vi "Set Node IDs.vi"(8 "error in (no error)":errorcluster, 10 "FolderIDs":T2, 11 "Station in":refnum<class "Station.lvclass">) -> (0 "error out":errorcluster, 3 "Station out":refnum<class "Station.lvclass">)   [LabVIEW 2021, in "Station.lvlib" / "Station.lvclass"]
uses:
  Station.lvclass
  <vilib>/OPCUA/controls/OPC UA Server Refnum.ctl
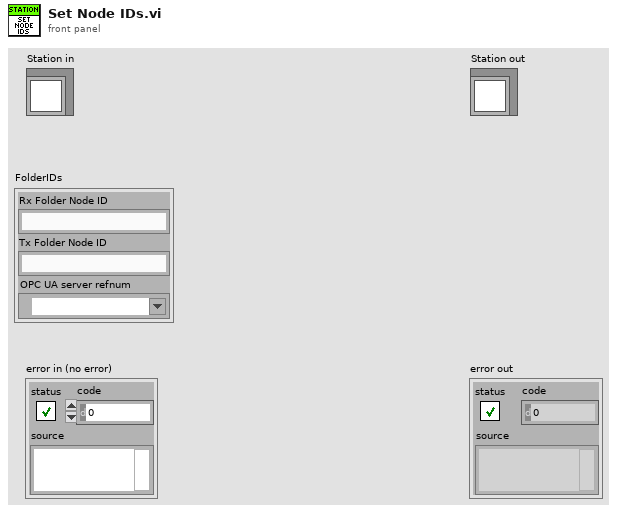
[diagram p1: front panel]
types:
  T1 = typedef "OPC UA Server Refnum.ctl" = refnum<k21>
  T2 = cluster{"Rx Folder Node ID":string, "Tx Folder Node ID":string, "OPC UA server refnum":T1}
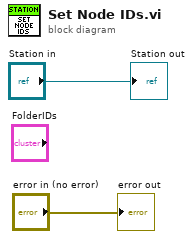
[diagram p0: block diagram]
diagram:
  "error out" <- "error in (no error)"
  "Station out" <- "Station in"
